vi "Chad Magic Voodoo 3.vi"() -> ()   [LabVIEW 2016]
panel:
  in  "Add Wire Feed... (%)":dbl=4.0
  in  "For Every... (mm)":dbl=0.2
  out "W trigger Y":dbl
  out "C trigger Y":dbl
  out "R trigger Y":dbl
  in  "Window Bead Trigger heights":dbl[](array[numeric])
  in  "Robot Bead Trigger heights":dbl[](array[numeric])
  in  "Center Bead Trigger heights":dbl[](array[numeric])
  out "Shutter Open":bool
  in  "base path":path=path "C:/Users/Mark/Desktop/BeadScan"
  in  "Write Code":bool
  out "Bead3 Size":i32
  out "Bead2 Size":i32
  out "Bead1 Size":i32
  in  "Tab Control":T1(tab)
  in  "Mark Target Bead Height":bool
  out "All Beads":cluster{dbl[], dbl[]}[](graph)
  out "Target Bead Height":dbl
  in  "Set Correction C":bool
  in  "Set Trigger Offset":dbl
  in  "Center Bead Corrections":dbl[](array[numeric])
  in  "Center Bead Trigger Positions":dbl[](array[numeric])
  out "Center Bead #1":cluster{dbl[], dbl[]}[](graph)
  out "Center Bead Trigger":dbl
  in  "Set Trigger Center":bool
  in  "Undo":bool
  out "Difference From Bead Height Setpoint C":dbl
  out "Recommended % Change\n in Wire Feed C":dbl
  in  "Set Correction R":bool
  in  "Set Trigger Offset 2":dbl
  out "Robot Bead #2":cluster{dbl[], dbl[]}[](graph)
  in  "Robot Bead Trigger Positions":dbl[](array[numeric])
  in  "Robot Bead Corrections":dbl[](array[numeric])
  out "Robot Bead Trigger":dbl
  in  "Set Trigger Robot":bool
  in  "Undo":bool
  out "Difference From Bead Height Setpoint R":dbl
  out "Recommended % Change\n in Wire Feed R":dbl
  in  "Set Correction W":bool
  in  "Set Trigger Offset 3":dbl
  out "Window Bead #3":cluster{dbl[], dbl[]}[](graph)
  in  "Window Bead Trigger Positions":dbl[](array[numeric])
  in  "Window Bead Corrections":dbl[](array[numeric])
  out "Window Bead Trigger":dbl
  in  "Set Trigger Window":bool
  in  "Undo":bool
  out "Difference From Bead Height Setpoint W":dbl
  out "Recommended % Change\n in Wire Feed W":dbl
  in  "stop":bool
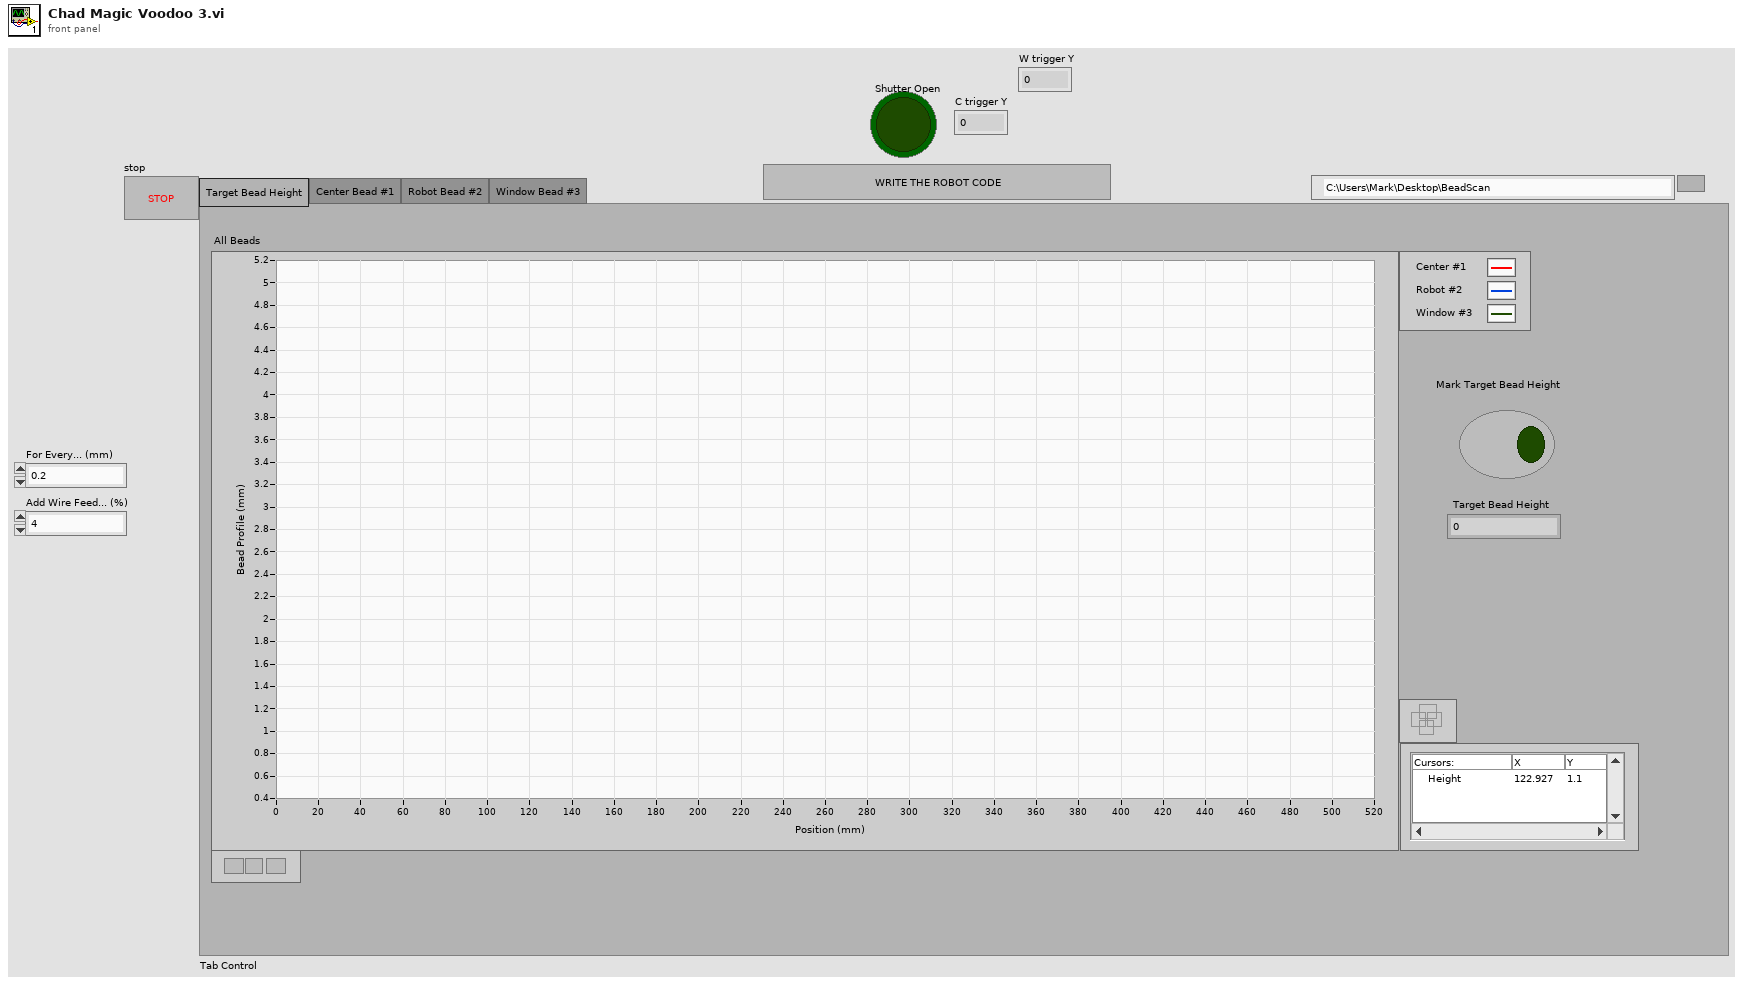
[diagram p1: front panel]
types:
  T1 = enum32{"Target Bead Height", "Center Bead #1", "Robot Bead #2", "Window Bead #3"}
  T2 = enum16{"open", "replace", "create", "open or create", "replace or create", "replace or create with confirmation"}
  T3 = cluster{"[0]":cluster{dbl[], dbl[]}, "[1]":cluster{dbl[], dbl[]}, "[2]":cluster{dbl[], dbl[]}}
  T4 = cluster{dbl[], "Center Bead Trigger heights":dbl[]}
  T5 = cluster{dbl[], "Window Bead Trigger heights":dbl[]}
  T6 = cluster{dbl[], "Robot Bead Trigger heights":dbl[]}
  T7 = cluster{dbl[], "Center Bead Trigger heights":dbl[]}[]
  T8 = cluster{dbl[], "Robot Bead Trigger heights":dbl[]}[]
  T9 = cluster{dbl[], "Window Bead Trigger heights":dbl[]}[]
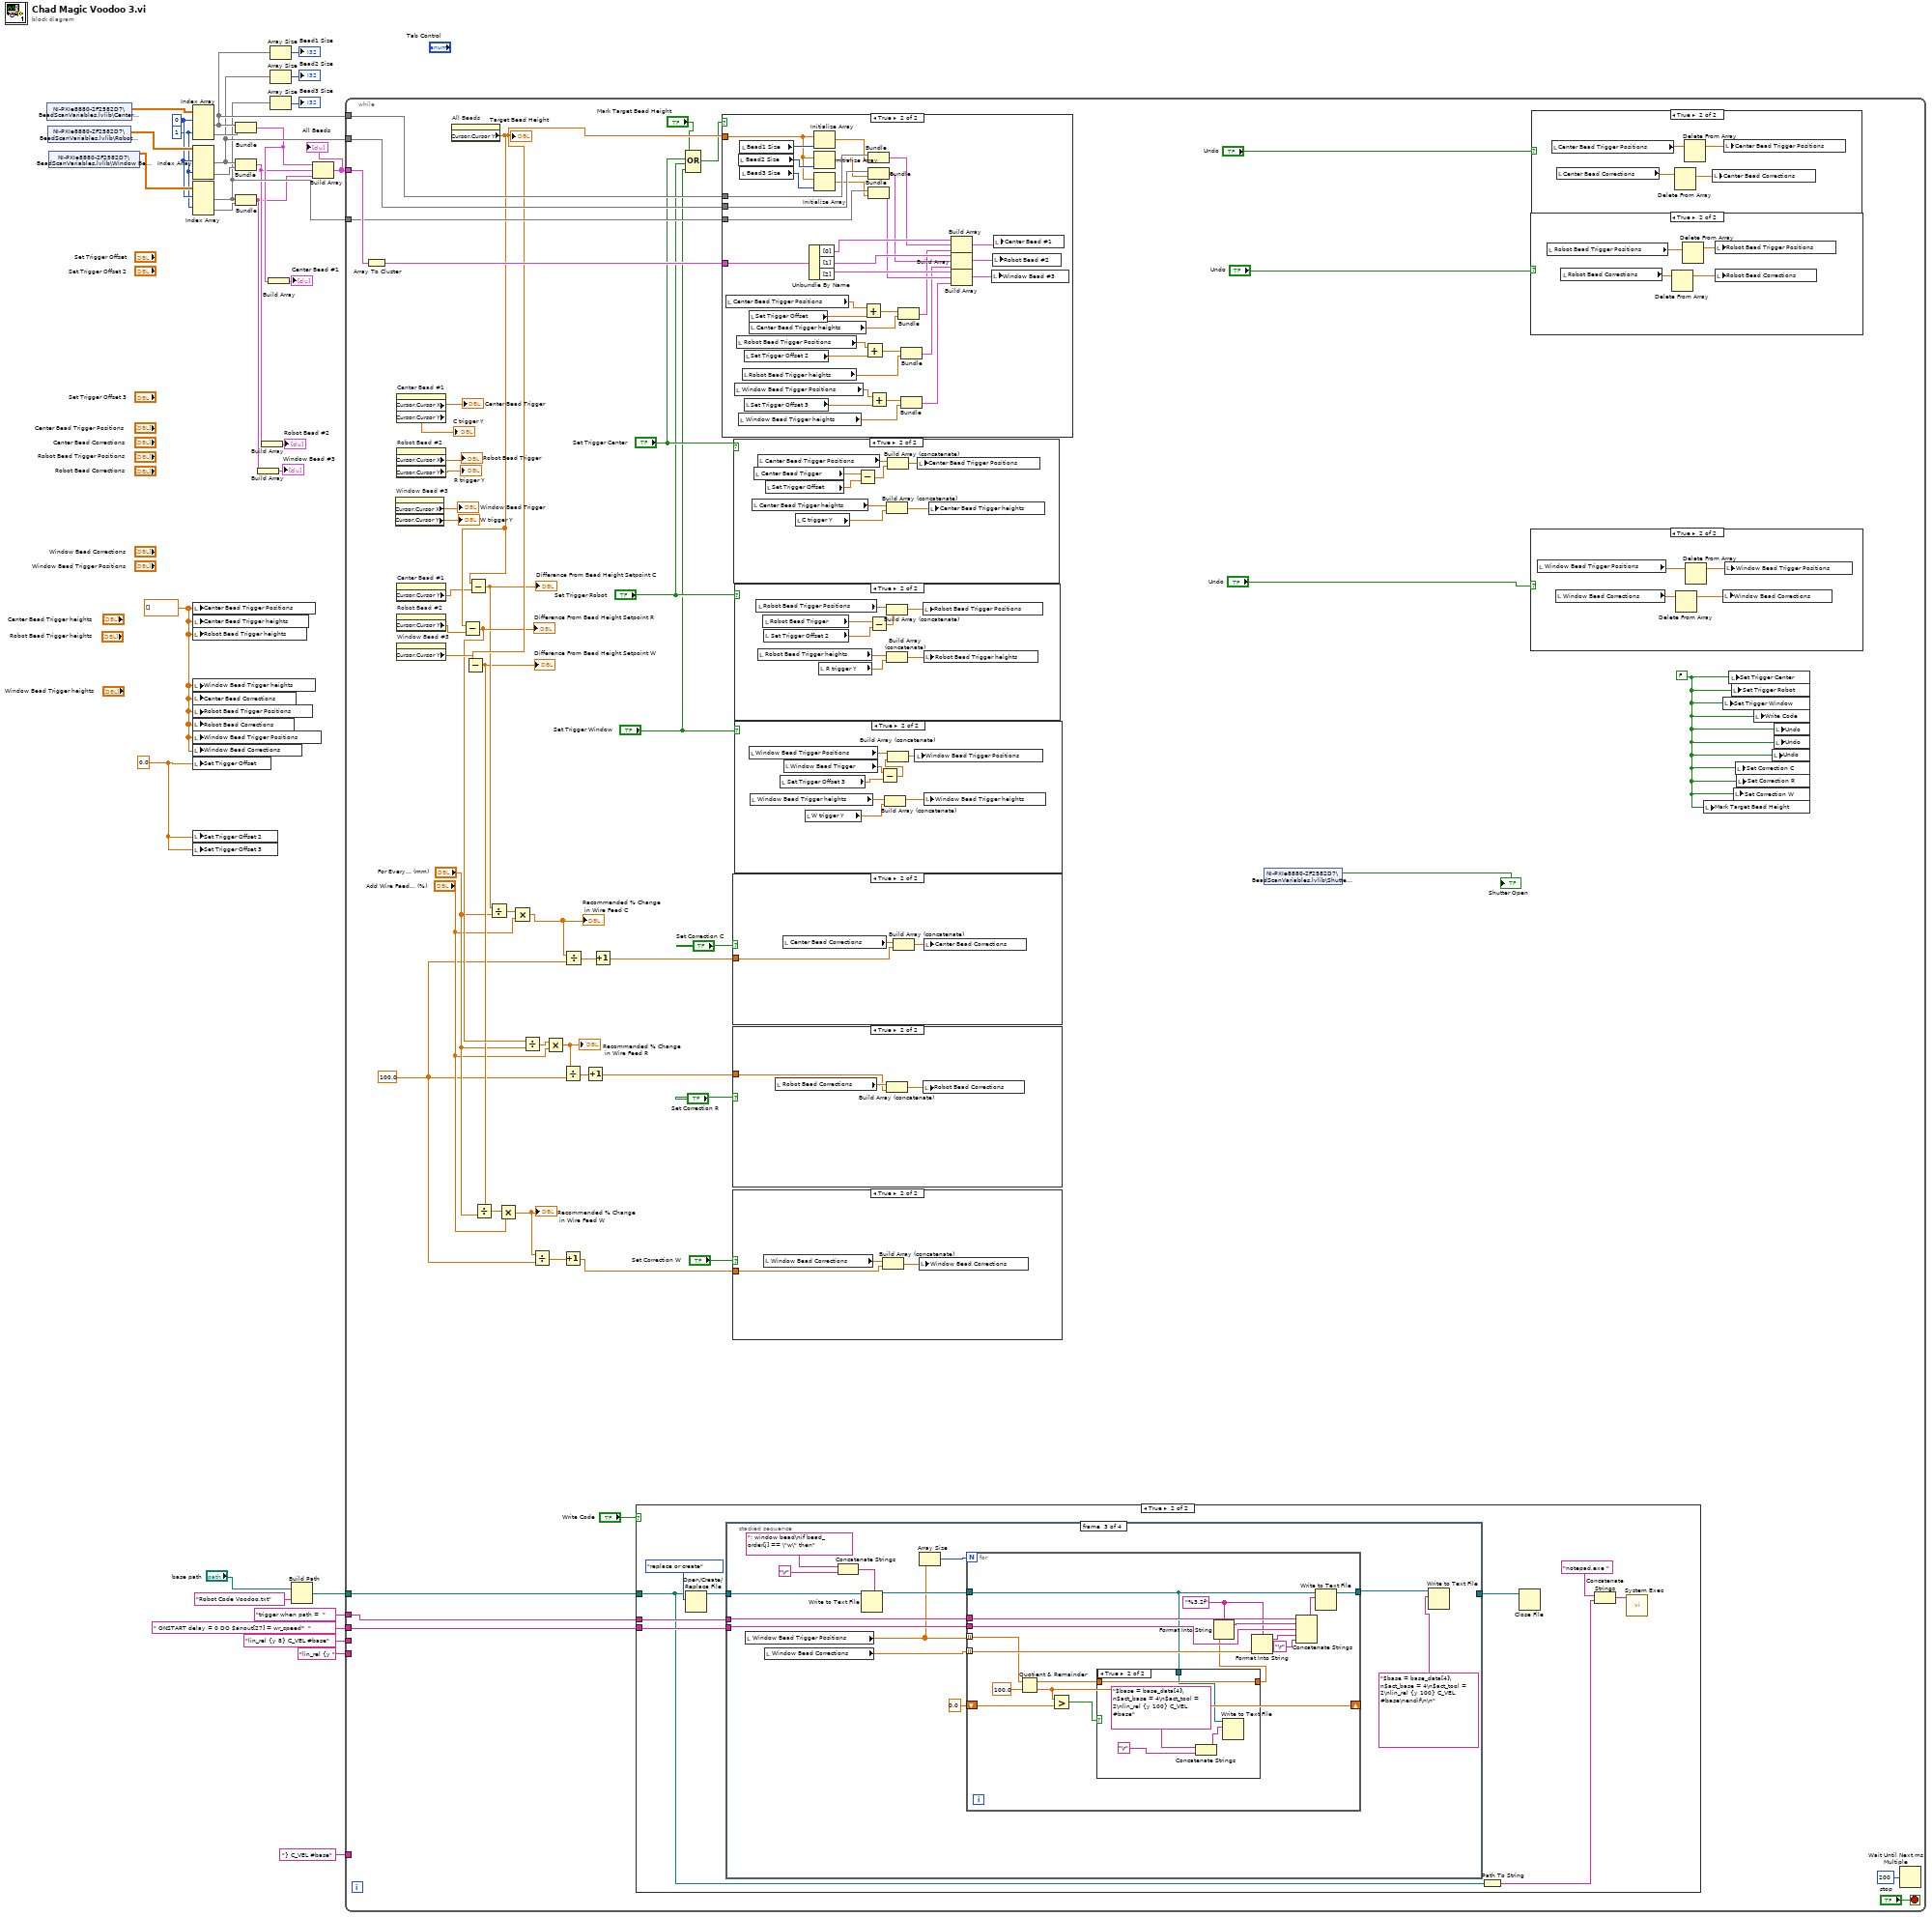
[diagram p0: block diagram]
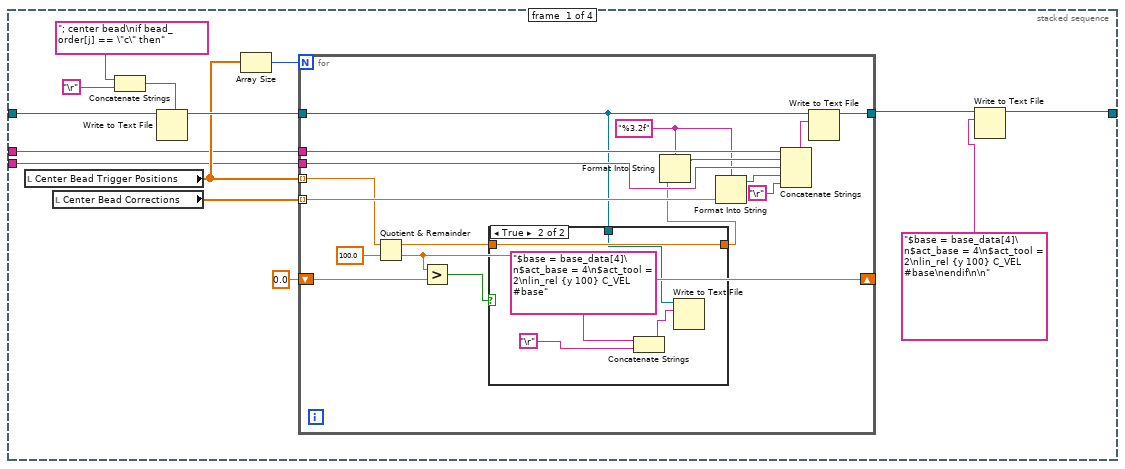
[diagram p6: hidden frame]
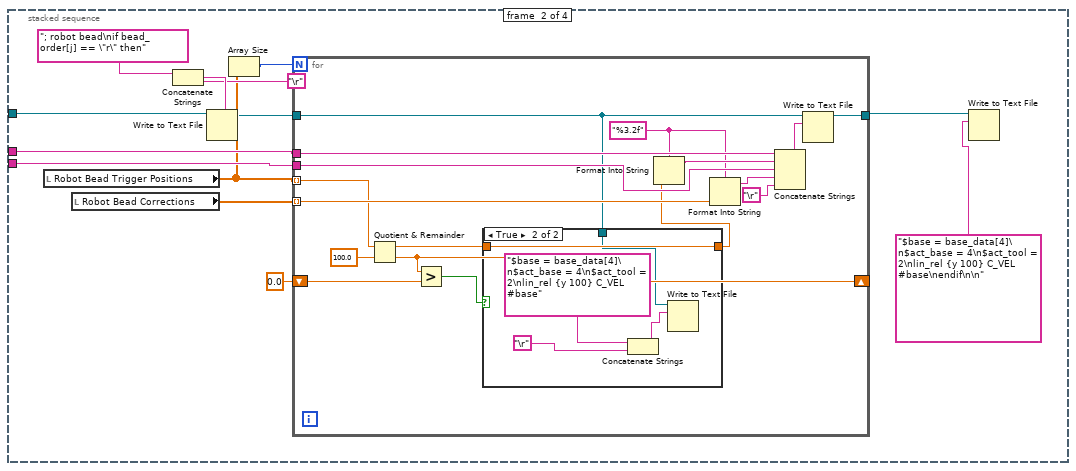
[diagram p8: hidden frame]
diagram:
  w2 = 0.0
  w1 = dbl[] []
  w26 = 1 ("index (row)")
  w27 = 0 ("index (row)")
  n1 = shared-variable "NI-PXIe8880-2F2582D7\\BeadScanVariables.lvlib\\Center Bead #1"() -> (w31:dbl[][])  [unwired: 1 in, 1 out]
  n2 = shared-variable "NI-PXIe8880-2F2582D7\\BeadScanVariables.lvlib\\Robot Bead #2"() -> (w29:dbl[][])  [unwired: 1 in, 1 out]
  n3 = shared-variable "NI-PXIe8880-2F2582D7\\BeadScanVariables.lvlib\\Window Bead #3"() -> (w28:dbl[][])  [unwired: 1 in, 1 out]
  n4 = Index Array(array=w31, index (row) #1=w27, index (row) #2=w26) -> (element #1=w19:dbl[], element #2=w30:dbl[])  [unwired: 2 in]
  n5 = Index Array(array=w29, index (row) #1=w27, index (row) #2=w26) -> (element #1=w18:dbl[], element #2=w25:dbl[])  [unwired: 2 in]
  n6 = Index Array(array=w28, index (row) #1=w27, index (row) #2=w26) -> (element #1=w17:dbl[], element #2=w24:dbl[])  [unwired: 2 in]
  n7 = local write "Center Bead Trigger Positions"(w1) -> ()
  n8 = local write "Center Bead Trigger heights"(w1) -> ()
  n9 = local write "Robot Bead Trigger heights"(w1) -> ()
  n10 = local write "Window Bead Trigger heights"(w1) -> ()
  n11 = local write "Center Bead Corrections"(w1) -> ()
  n12 = local write "Robot Bead Trigger Positions"(w1) -> ()
  n13 = local write "Robot Bead Corrections"(w1) -> ()
  n14 = local write "Window Bead Trigger Positions"(w1) -> ()
  n15 = local write "Window Bead Corrections"(w1) -> ()
  n16 = local write "Set Trigger Offset"(w2) -> ()
  n17 = local write "Set Trigger Offset 2"(w2) -> ()
  n18 = local write "Set Trigger Offset 3"(w2) -> ()
  n19 = Bundle(w18, w25) -> (w14:cluster{dbl[], dbl[]})  [unwired: 1 in]
  n20 = Bundle(w19, w30) -> (w15:cluster{dbl[], dbl[]})  [unwired: 1 in]
  n21 = Bundle(w17, w24) -> (w11:cluster{dbl[], dbl[]})  [unwired: 1 in]
  n22 = Build Array(w11) -> (→"Window Bead #3":cluster{dbl[], dbl[]}[])
  n23 = Build Array(w14) -> (→"Robot Bead #2":cluster{dbl[], dbl[]}[])
  n24 = Build Array(w15) -> (→"Center Bead #1":cluster{dbl[], dbl[]}[])
  n25 = Array Size(array=w19) -> (size(s)=→"Bead1 Size":i32)
  n26 = Array Size(array=w18) -> (size(s)=→"Bead2 Size":i32)
  n27 = Array Size(array=w17) -> (size(s)=→"Bead3 Size":i32)
  n28 = Build Path(base path="base path", name or relative path="Robot Code Voodoo.txt") -> (appended path=w8:path)
  n29 = Build Array(w15, w14, w11) -> (w20:cluster{dbl[], dbl[]}[])
  "All Beads" <- w20
  n30 = while {
    tunnel: w20 -> [w80]
    tunnel: w19 -> [w78]
    tunnel: w18 -> [w77]
    tunnel: w17 -> [w76]
    tunnel: w8 -> [w71]
    tunnel: "trigger when path =  " -> [w70]
    tunnel: " ONSTART delay = 0 DO $anout[27] = wr_speed*  " -> [w69]
    tunnel: "lin_rel {y 8} C_VEL #base" -> [_]
    tunnel: "lin_rel {y " -> [_]
    tunnel: "} C_VEL #base" -> [_]
    stop <- "stop" stop-if-true
    w39 = 100.0 ("y")
    w32 = FALSE
    n31 = Array To Cluster(array=w80) -> (cluster=w79:T3)
    n32 = property on="Window Bead #3" class="XYGraph (strict)"() -> ("Cursor.Cursor X"=→"Window Bead Trigger":dbl, "Cursor.Cursor Y"=→"W trigger Y":dbl)  [unwired: 2 in, 2 out]
    n33 = property on="Center Bead #1" class="XYGraph (strict)"() -> ("Cursor.Cursor X"=→"Center Bead Trigger":dbl, "Cursor.Cursor Y"=→"C trigger Y":dbl)  [unwired: 2 in, 2 out]
    n34 = property on="Robot Bead #2" class="XYGraph (strict)"() -> ("Cursor.Cursor X"=→"Robot Bead Trigger":dbl, "Cursor.Cursor Y"=→"R trigger Y":dbl)  [unwired: 2 in, 2 out]
    n35 = property on="Center Bead #1" class="XYGraph (strict)"() -> ("Cursor.Cursor Y"=w65:dbl)  [unwired: 2 in, 2 out]
    n36 = property on="Robot Bead #2" class="XYGraph (strict)"() -> ("Cursor.Cursor Y"=w64:dbl)  [unwired: 2 in, 2 out]
    n37 = property on="Window Bead #3" class="XYGraph (strict)"() -> ("Cursor.Cursor Y"=w63:dbl)  [unwired: 2 in, 2 out]
    n38 = property on="All Beads" class="XYGraph (strict)"() -> ("Cursor.Cursor Y"=w66:dbl)  [unwired: 2 in, 2 out]
    "Target Bead Height" <- w66
    n39 = Subtract(x=w66, y=w64) -> (x-y=w51:dbl)
    "Difference From Bead Height Setpoint R" <- w51
    n40 = Subtract(x=w66, y=w63) -> (x-y=w48:dbl)
    "Difference From Bead Height Setpoint W" <- w48
    n41 = Subtract(x=w66, y=w65) -> (x-y=w49:dbl)
    "Difference From Bead Height Setpoint C" <- w49
    n42 = Divide(x=w48, y="For Every... (mm)") -> (x/y=w52:dbl)
    n43 = Divide(x=w49, y="For Every... (mm)") -> (x/y=w50:dbl)
    n44 = Multiply(x=w52, y="Add Wire Feed... (%)") -> (x*y=w40:dbl)
    "Recommended % Change\n in Wire Feed W" <- w40
    n45 = Multiply(x=w50, y="Add Wire Feed... (%)") -> (x*y=w41:dbl)
    "Recommended % Change\n in Wire Feed C" <- w41
    n46 = Divide(x=w51, y="For Every... (mm)") -> (x/y=w53:dbl)
    n47 = Divide(x=w40, y=w39) -> (x/y=w36:dbl)
    n48 = Multiply(x=w53, y="Add Wire Feed... (%)") -> (x*y=w42:dbl)
    "Recommended % Change\n in Wire Feed R" <- w42
    n49 = Divide(x=w42, y=w39) -> (x/y=w38:dbl)
    n50 = Increment(x=w36) -> (x+1=w35:dbl)
    n51 = Divide(x=w41, y=w39) -> (x/y=w37:dbl)
    n52 = Increment(x=w38) -> (x+1=w34:dbl)
    n53 = Increment(x=w37) -> (x+1=w33:dbl)
    n54 = case shown="True" "Write Code" {
      tunnel: w71 -> [_ w93]
      tunnel: w70 -> [_ w100]
      tunnel: w69 -> [_ w99]
      frame False {
      }
      frame True {
        n55 = Open/Create/Replace File(file path (use dialog)=w93, operation (0:open)=T2."replace or create") -> (refnum out=w101:refnum<file>)  [unwired: 4 in, 2 out]
        n56 = stacked-sequence {
          tunnel: w101 -> [w112 w149 w185 _]
          tunnel: w100 -> [w107 w144 w178 _]
          tunnel: w99 -> [w106 w143 w177 _]
          tunnel: [w103 _ _ _] -> w98
          frame #0 {
            n57 = local read "Center Bead Trigger Positions"() -> (w109:dbl[])
            n58 = local read "Center Bead Corrections"() -> (w108:dbl[])
            n59 = Concatenate Strings("; center bead\nif bead_order[j] == \"c\" then", "\r") -> (w113:string)
            n60 = Write to Text File(file (use dialog)=w112, text=w113) -> (refnum out=w111:refnum<file>)  [unwired: 2 in, 2 out]
            n61 = Array Size(array=w109) -> (size(s)=w110:i32)
            n62 = for {
              N: w110 -> [_]
              tunnel: w111 -> [w116]
              tunnel: w109 -> [w123] mode=indexing
              tunnel: w108 -> [w128] mode=indexing
              tunnel: w107 -> [w132]
              tunnel: w106 -> [w129]
              tunnel: [w126] -> w104
              shift-right: [w121] -> _
              shift-left: 0.0 -> [w120]
              w125 = "%3.2f" ("format string")
              n63 = Quotient & Remainder(x=w123, y=100.0) -> (x-y*floor(x/y)=w118:dbl, floor(x/y)=w121:dbl)
              n64 = Greater?(x=w121, y=w120) -> (0:w119:bool)
              n65 = case shown="True" w119 {
                tunnel: w118 -> [w133 w138]
                tunnel: [w133 w138] -> w117
                tunnel: w116 -> [_ w137]
                frame False {
                }
                frame True {
                  n66 = Concatenate Strings("$base = base_data[4]\n$act_base = 4\n$act_tool = 2\nlin_rel {y 100} C_VEL #base", "\r") -> (w134:string)
                  n67 = Write to Text File(file (use dialog)=w137, text=w134) -> ()  [unwired: 2 in, 3 out]
                }
              }
              n68 = Format Into String(format string=w125, w117) -> (resulting string=w131:string)  [unwired: 2 in, 1 out]
              n69 = Format Into String(format string=w125, w128) -> (resulting string=w127:string)  [unwired: 2 in, 1 out]
              n70 = Concatenate Strings(w132, w131, w129, w127, "\r") -> (w130:string)
              n71 = Write to Text File(file (use dialog)=w116, text=w130) -> (refnum out=w126:refnum<file>)  [unwired: 2 in, 2 out]
            }
            n72 = Write to Text File(file (use dialog)=w104, text="$base = base_data[4]\n$act_base = 4\n$act_tool = 2\nlin_rel {y 100} C_VEL #base\nendif\n\n") -> (refnum out=w103:refnum<file>)  [unwired: 2 in, 2 out]
          }
          frame #1 {
            n73 = local read "Robot Bead Trigger Positions"() -> (w142:dbl[])
            n74 = local read "Robot Bead Corrections"() -> (w141:dbl[])
            n75 = Concatenate Strings("; robot bead\nif bead_order[j] == \"r\" then", "\r") -> (w150:string)
            n76 = Write to Text File(file (use dialog)=w149, text=w150) -> (refnum out=w140:refnum<file>)  [unwired: 2 in, 2 out]
            n77 = Array Size(array=w142) -> (size(s)=w139:i32)
            n78 = for {
              N: w139 -> [_]
              tunnel: w140 -> [w152]
              tunnel: w142 -> [w159] mode=indexing
              tunnel: w141 -> [w164] mode=indexing
              tunnel: w144 -> [w168]
              tunnel: w143 -> [w165]
              tunnel: [w162] -> w146
              shift-right: [w157] -> _
              shift-left: 0.0 -> [w156]
              w161 = "%3.2f" ("format string")
              n79 = Quotient & Remainder(x=w159, y=100.0) -> (x-y*floor(x/y)=w154:dbl, floor(x/y)=w157:dbl)
              n80 = Greater?(x=w157, y=w156) -> (0:w155:bool)
              n81 = case shown="True" w155 {
                tunnel: w154 -> [w169 w174]
                tunnel: [w169 w174] -> w153
                tunnel: w152 -> [_ w173]
                frame False {
                }
                frame True {
                  n82 = Concatenate Strings("$base = base_data[4]\n$act_base = 4\n$act_tool = 2\nlin_rel {y 100} C_VEL #base", "\r") -> (w170:string)
                  n83 = Write to Text File(file (use dialog)=w173, text=w170) -> ()  [unwired: 2 in, 3 out]
                }
              }
              n84 = Format Into String(format string=w161, w153) -> (resulting string=w167:string)  [unwired: 2 in, 1 out]
              n85 = Format Into String(format string=w161, w164) -> (resulting string=w163:string)  [unwired: 2 in, 1 out]
              n86 = Concatenate Strings(w168, w167, w165, w163, "\r") -> (w166:string)
              n87 = Write to Text File(file (use dialog)=w152, text=w166) -> (refnum out=w162:refnum<file>)  [unwired: 2 in, 2 out]
            }
            n88 = Write to Text File(file (use dialog)=w146, text="$base = base_data[4]\n$act_base = 4\n$act_tool = 2\nlin_rel {y 100} C_VEL #base\nendif\n\n") -> ()  [unwired: 2 in, 3 out]
          }
          frame #2 {
            n89 = local read "Window Bead Trigger Positions"() -> (w176:dbl[])
            n90 = local read "Window Bead Corrections"() -> (w175:dbl[])
            n91 = Concatenate Strings("; window bead\nif bead_order[j] == \"w\" then", "\r") -> (w186:string)
            n92 = Write to Text File(file (use dialog)=w185, text=w186) -> (refnum out=w179:refnum<file>)  [unwired: 2 in, 2 out]
            n93 = Array Size(array=w176) -> (size(s)=w180:i32)
            n94 = for {
              N: w180 -> [_]
              tunnel: w179 -> [w188]
              tunnel: w176 -> [w195] mode=indexing
              tunnel: w175 -> [w200] mode=indexing
              tunnel: w178 -> [w204]
              tunnel: w177 -> [w201]
              tunnel: [w198] -> w182
              shift-right: [w193] -> _
              shift-left: 0.0 -> [w192]
              w197 = "%3.2f" ("format string")
              n95 = Quotient & Remainder(x=w195, y=100.0) -> (x-y*floor(x/y)=w190:dbl, floor(x/y)=w193:dbl)
              n96 = Greater?(x=w193, y=w192) -> (0:w191:bool)
              n97 = case shown="True" w191 {
                tunnel: w190 -> [w205 w210]
                tunnel: [w205 w210] -> w189
                tunnel: w188 -> [_ w209]
                frame False {
                }
                frame True {
                  n98 = Concatenate Strings("$base = base_data[4]\n$act_base = 4\n$act_tool = 2\nlin_rel {y 100} C_VEL #base", "\r") -> (w206:string)
                  n99 = Write to Text File(file (use dialog)=w209, text=w206) -> ()  [unwired: 2 in, 3 out]
                }
              }
              n100 = Format Into String(format string=w197, w189) -> (resulting string=w203:string)  [unwired: 2 in, 1 out]
              n101 = Format Into String(format string=w197, w200) -> (resulting string=w199:string)  [unwired: 2 in, 1 out]
              n102 = Concatenate Strings(w204, w203, w201, w199, "\r") -> (w202:string)
              n103 = Write to Text File(file (use dialog)=w188, text=w202) -> (refnum out=w198:refnum<file>)  [unwired: 2 in, 2 out]
            }
            n104 = Write to Text File(file (use dialog)=w182, text="$base = base_data[4]\n$act_base = 4\n$act_tool = 2\nlin_rel {y 100} C_VEL #base\nendif\n\n") -> ()  [unwired: 2 in, 3 out]
          }
          frame #3 {
          }
        }
        n105 = Path To String(path=w93) -> (string=w94:string)
        n106 = Close File(refnum=w98) -> ()  [unwired: 1 in, 2 out]
        n107 = Concatenate Strings("notepad.exe " ("command line"), w94) -> (w96:string)
        n108 = call <vilib>:"System Exec.vi"("command line"=w96) -> ()  [unwired: 7 in, 4 out]
      }
    }
    n109 = Compound Arithmetic op=OR("Mark Target Bead Height", "Set Trigger Center", "Set Trigger Robot", "Set Trigger Window") -> (w57:bool)
    n110 = case shown="True" w57 {
      tunnel: w66 -> [_ w279]
      tunnel: w79 -> [_ w277]
      tunnel: w78 -> [_ w276]
      tunnel: w77 -> [_ w274]
      tunnel: w76 -> [_ w273]
      frame False {
      }
      frame True {
        n111 = local read "Center Bead Trigger Positions"() -> (w257:dbl[])
        n112 = local read "Window Bead Trigger Positions"() -> (w251:dbl[])
        n113 = local read "Robot Bead Trigger Positions"() -> (w254:dbl[])
        n114 = local read "Bead2 Size"() -> (w280:i32)
        n115 = local read "Window Bead Trigger heights"() -> (w250:dbl[])
        n116 = local read "Bead1 Size"() -> (w281:i32)
        n117 = local read "Bead3 Size"() -> (w278:i32)
        n118 = local read "Robot Bead Trigger heights"() -> (w252:dbl[])
        n119 = local read "Set Trigger Offset 2"() -> (w260:dbl)
        n120 = local read "Set Trigger Offset 3"() -> (w259:dbl)
        n121 = local read "Set Trigger Offset"() -> (w261:dbl)
        n122 = local read "Center Bead Trigger heights"() -> (w255:dbl[])
        n123 = Unbundle By Name(w277) -> ("[0]"=w270:cluster{dbl[], dbl[]}, "[1]"=w268:cluster{dbl[], dbl[]}, "[2]"=w266:cluster{dbl[], dbl[]})
        n124 = Initialize Array(w279, w281) -> (w275:dbl[])
        n125 = Initialize Array(w279, w280) -> (w271:dbl[])
        n126 = Initialize Array(w279, w278) -> (w272:dbl[])
        n127 = Add(x=w257, y=w261) -> (x+y=w256:dbl[])
        n128 = Add(x=w254, y=w260) -> (x+y=w253:dbl[])
        n129 = Bundle(w276, w275) -> (w269:cluster{dbl[], dbl[]})  [unwired: 1 in]
        n130 = Bundle(w274, w271) -> (w267:cluster{dbl[], dbl[]})  [unwired: 1 in]
        n131 = Bundle(w273, w272) -> (w265:cluster{dbl[], dbl[]})  [unwired: 1 in]
        n132 = Add(x=w251, y=w259) -> (x+y=w258:dbl[])
        n133 = Bundle(w256, "Center Bead Trigger heights"=w255) -> (w249:T4)  [unwired: 1 in]
        n134 = Bundle(w258, "Window Bead Trigger heights"=w250) -> (w247:T5)  [unwired: 1 in]
        n135 = Bundle(w253, "Robot Bead Trigger heights"=w252) -> (w248:T6)  [unwired: 1 in]
        n136 = Build Array(w270, w269, w249) -> (w264:T7)
        n137 = Build Array(w268, w267, w248) -> (w263:T8)
        n138 = Build Array(w266, w265, w247) -> (w262:T9)
        n139 = local write "Window Bead #3"(w262) -> ()
        n140 = local write "Robot Bead #2"(w263) -> ()
        n141 = local write "Center Bead #1"(w264) -> ()
      }
    }
    n142 = case shown="True" "Set Correction C" {
      tunnel: w33 -> [_ w90]
      frame False {
      }
      frame True {
        n143 = local read "Center Bead Corrections"() -> (w92:dbl[])
        n144 = Build Array (concatenate)(w92, w90) -> (w91:dbl[])
        n145 = local write "Center Bead Corrections"(w91) -> ()
      }
    }
    n146 = case shown="True" "Set Correction R" {
      tunnel: w34 -> [_ w87]
      frame False {
      }
      frame True {
        n147 = local read "Robot Bead Corrections"() -> (w89:dbl[])
        n148 = Build Array (concatenate)(w89, w87) -> (w88:dbl[])
        n149 = local write "Robot Bead Corrections"(w88) -> ()
      }
    }
    n150 = case shown="True" "Set Correction W" {
      tunnel: w35 -> [_ w84]
      frame False {
      }
      frame True {
        n151 = local read "Window Bead Corrections"() -> (w86:dbl[])
        n152 = Build Array (concatenate)(w86, w84) -> (w85:dbl[])
        n153 = local write "Window Bead Corrections"(w85) -> ()
      }
    }
    n154 = case shown="True" "Set Trigger Center" {
      frame False {
      }
      frame True {
        n155 = local read "Center Bead Trigger heights"() -> (w241:dbl[])
        n156 = local read "Center Bead Trigger"() -> (w244:dbl)
        n157 = local read "Center Bead Trigger Positions"() -> (w246:dbl[])
        n158 = local read "Set Trigger Offset"() -> (w242:dbl)
        n159 = local read "C trigger Y"() -> (w240:dbl)
        n160 = Subtract(x=w244, y=w242) -> (x-y=w243:dbl)
        n161 = Build Array (concatenate)(w241, w240) -> (w239:dbl[])
        n162 = Build Array (concatenate)(w246, w243) -> (w245:dbl[])
        n163 = local write "Center Bead Trigger Positions"(w245) -> ()
        n164 = local write "Center Bead Trigger heights"(w239) -> ()
      }
    }
    n165 = case shown="True" "Set Trigger Robot" {
      frame False {
      }
      frame True {
        n166 = local read "Robot Bead Trigger Positions"() -> (w238:dbl[])
        n167 = local read "Robot Bead Trigger heights"() -> (w232:dbl[])
        n168 = local read "Robot Bead Trigger"() -> (w236:dbl)
        n169 = local read "Set Trigger Offset 2"() -> (w234:dbl)
        n170 = local read "R trigger Y"() -> (w231:dbl)
        n171 = Subtract(x=w236, y=w234) -> (x-y=w235:dbl)
        n172 = Build Array (concatenate)(w232, w231) -> (w233:dbl[])
        n173 = Build Array (concatenate)(w238, w235) -> (w237:dbl[])
        n174 = local write "Robot Bead Trigger Positions"(w237) -> ()
        n175 = local write "Robot Bead Trigger heights"(w233) -> ()
      }
    }
    n176 = case shown="True" "Set Trigger Window" {
      frame False {
      }
      frame True {
        n177 = local read "Window Bead Trigger Positions"() -> (w230:dbl[])
        n178 = local read "Window Bead Trigger heights"() -> (w225:dbl[])
        n179 = local read "Set Trigger Offset 3"() -> (w228:dbl)
        n180 = local read "Window Bead Trigger"() -> (w227:dbl)
        n181 = local read "W trigger Y"() -> (w224:dbl)
        n182 = Subtract(x=w227, y=w228) -> (x-y=w226:dbl)
        n183 = Build Array (concatenate)(w225, w224) -> (w223:dbl[])
        n184 = Build Array (concatenate)(w230, w226) -> (w229:dbl[])
        n185 = local write "Window Bead Trigger Positions"(w229) -> ()
        n186 = local write "Window Bead Trigger heights"(w223) -> ()
      }
    }
    n187 = shared-variable "NI-PXIe8880-2F2582D7\\BeadScanVariables.lvlib\\Shutter Open"() -> (→"Shutter Open":bool)  [unwired: 1 in, 1 out]
    n188 = case shown="True" "Undo" {
      frame False {
      }
      frame True {
        n189 = local read "Robot Bead Trigger Positions"() -> (w217:dbl[])
        n190 = local read "Robot Bead Corrections"() -> (w218:dbl[])
        n191 = Delete From Array(array=w218) -> (array with subset deleted=w215:dbl[])  [unwired: 2 in, 1 out]
        n192 = Delete From Array(array=w217) -> (array with subset deleted=w216:dbl[])  [unwired: 2 in, 1 out]
        n193 = local write "Robot Bead Trigger Positions"(w216) -> ()
        n194 = local write "Robot Bead Corrections"(w215) -> ()
      }
    }
    n195 = case shown="True" "Undo" {
      frame False {
      }
      frame True {
        n196 = local read "Window Bead Trigger Positions"() -> (w213:dbl[])
        n197 = local read "Window Bead Corrections"() -> (w212:dbl[])
        n198 = Delete From Array(array=w212) -> (array with subset deleted=w211:dbl[])  [unwired: 2 in, 1 out]
        n199 = Delete From Array(array=w213) -> (array with subset deleted=w214:dbl[])  [unwired: 2 in, 1 out]
        n200 = local write "Window Bead Corrections"(w211) -> ()
        n201 = local write "Window Bead Trigger Positions"(w214) -> ()
      }
    }
    n202 = case shown="True" "Undo" {
      frame False {
      }
      frame True {
        n203 = local read "Center Bead Trigger Positions"() -> (w221:dbl[])
        n204 = local read "Center Bead Corrections"() -> (w220:dbl[])
        n205 = Delete From Array(array=w220) -> (array with subset deleted=w219:dbl[])  [unwired: 2 in, 1 out]
        n206 = Delete From Array(array=w221) -> (array with subset deleted=w222:dbl[])  [unwired: 2 in, 1 out]
        n207 = local write "Center Bead Corrections"(w219) -> ()
        n208 = local write "Center Bead Trigger Positions"(w222) -> ()
      }
    }
    n209 = local write "Mark Target Bead Height"(w32) -> ()
    n210 = local write "Set Trigger Window"(w32) -> ()
    n211 = local write "Set Trigger Center"(w32) -> ()
    n212 = local write "Set Trigger Robot"(w32) -> ()
    n213 = local write "Set Correction W"(w32) -> ()
    n214 = local write "Set Correction C"(w32) -> ()
    n215 = local write "Set Correction R"(w32) -> ()
    n216 = local write "Write Code"(w32) -> ()
    n217 = local write "Undo"(w32) -> ()
    n218 = local write "Undo"(w32) -> ()
    n219 = local write "Undo"(w32) -> ()
    n220 = Wait Until Next ms Multiple(millisecond multiple=u32 200) -> ()  [unwired: 1 out]
  }
